vi "Mode (Set).vi"(6 "ISOBUS address":T4=-1 caption="ISOBUS address (-1)", 8 "error in":errorcluster, 9 "Password":string, 10 "Mode":T1="NORM" caption="User Mode", 11 "Mercury Reference In":T5) -> (0 "error out":errorcluster, 2 "Response":T3, 3 "Mercury Reference Out":T5, 4 "Valid?":T2)   [LabVIEW 2014, in "Mercury iXX.lvlib" / "System.lvlib"]
doc: "Set the current user mode according to the instrument."
uses:
  System.lvlib
  Controls/Mercury Reference.ctl
  Controls/Comms Transport Layer.ctl
  Private/Controls/Query Dynamic Reference.ctl
  Controls/ISOBus Address.ctl
  Controls/Response String.ctl
  Controls/Is Valid LED.ctl
  Controls/User Mode.ctl
  Mercury iXX.lvlib
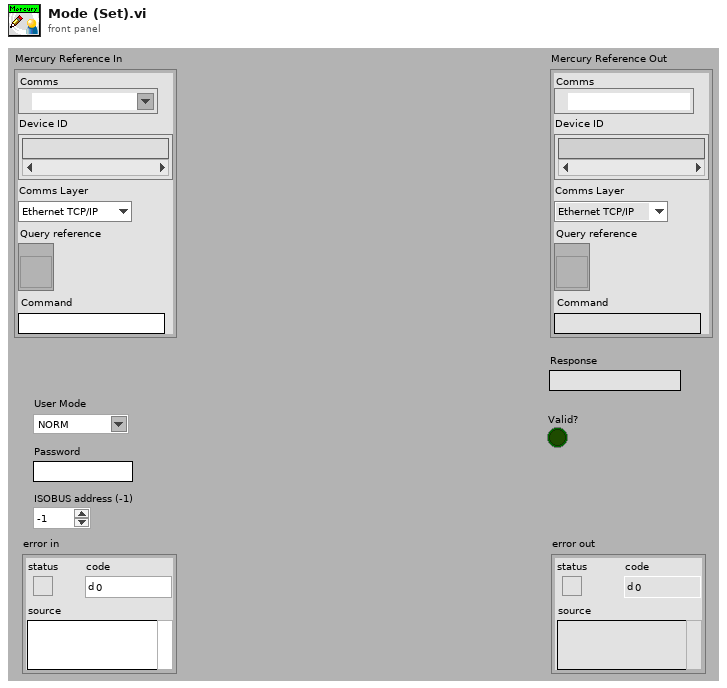
[diagram p1: front panel]
types:
  T1 = typedef "Mercury iXX.lvlib/System.lvlib/User Mode.ctl" = string
  T2 = typedef "Mercury iXX.lvlib/Is Valid LED.ctl" = bool
  T3 = typedef "Mercury iXX.lvlib/Response String.ctl" = string
  T4 = typedef "Mercury iXX.lvlib/ISOBus Address.ctl" = i32
  T5 = typedef "Mercury iXX.lvlib/Mercury Reference.ctl" = cluster{"Comms":refnum<visa-resource-name>, "Device ID":string[], "Comms Layer":T6, "Command":string, "Query reference":T7}
  T6 = typedef "Mercury iXX.lvlib/Comms Transport Layer.ctl" = enum16{"Ethernet TCP/IP", "USB", "ISOBus - RS-232", "GPIB"}
  T7 = typedef "Mercury iXX.lvlib/Query Dynamic Reference.ctl" = refnum<vi>
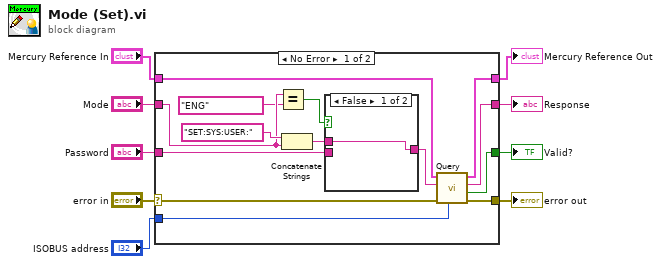
[diagram p0: block diagram]
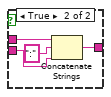
[diagram p2: hidden frame]
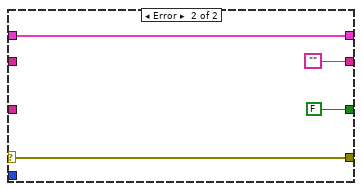
[diagram p3: hidden frame]
diagram:
  n1 = case shown="No Error" "error in" {
    selector: "error in" -> [w20 w31]
    tunnel: "Mercury Reference In" -> [w23 w32]
    tunnel: [w21 w32] -> w8
    tunnel: [w22 w31] -> w7
    tunnel: "ISOBUS address" -> [w19 _]
    tunnel: [w17 ""] -> w4
    tunnel: "Mode" -> [w15 _]
    tunnel: [w16 FALSE ("Valid?")] -> w3
    tunnel: "Password" -> [w11 _]
    frame No Error {
      n2 = Equal?(x=w15, y=T1 "ENG") -> (x = y?=w13:bool)
      n3 = Concatenate Strings("SET:SYS:USER:" ("Command"), w15) -> (w12:string)
      n4 = case shown="False" w13 {
        tunnel: w12 -> [w24 w28]
        tunnel: w11 -> [_ w26]
        tunnel: [w24 w25] -> w10
        frame False {
        }
        frame True {
          n5 = Concatenate Strings(w28, ":" ("Command"), w26) -> (w25:string)
        }
      }
      n6 = call "Query.vi"("ISOBUS address"=w19, "error in"=w20, "Command"=w10, "Mercury Reference In"=w23) -> ("error out"=w22:errorcluster, "Valid?"=w16:bool, "Data"=w17:string, "Mercury Reference Out"=w21:T5)  [unwired: 1 in, 3 out]
    }
    frame Error {
    }
  }
  "Mercury Reference Out" <- w8
  "error out" <- w7
  "Response" <- w4
  "Valid?" <- w3
